vi "modSingle.vi"(0 "signal":fxp<+,18,0>, 1 "Parameters":T1, 2 "Enable":bool, 11 "triangleOffset":fxp<+,19,1>) -> (4 "output":T2)   [LabVIEW 2017, in "BuckBoost.lvlib"]
uses:
  BuckBoost.lvlib
  modOutput.ctl
  modParameters.ctl
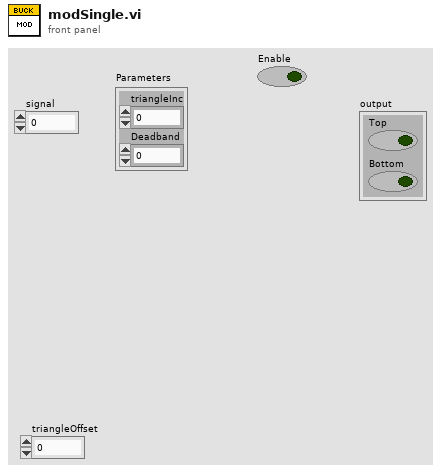
[diagram p1: front panel]
types:
  T1 = typedef "BuckBoost.lvlib/modParameters.ctl" = cluster{"triangleInc":fxp<+,18,0>, "Deadband":u16}
  T2 = typedef "BuckBoost.lvlib/modOutput.ctl" = cluster{"Top":bool, "Bottom":bool}
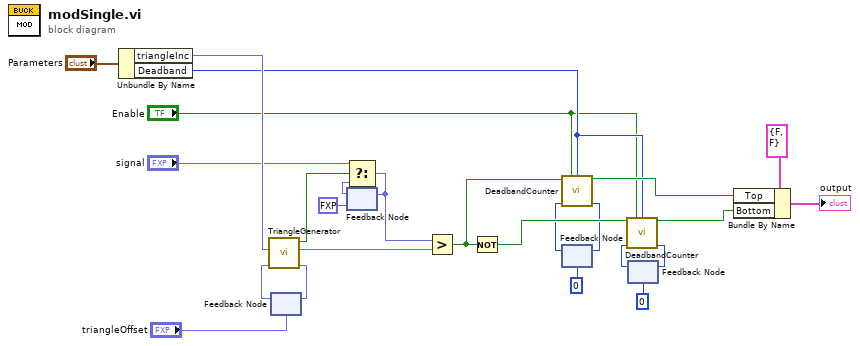
[diagram p0: block diagram]
diagram:
  n1 = Unbundle By Name("Parameters") -> ("triangleInc"=w17:fxp<+,18,0>, "Deadband"=w16:u16)
  n2 = feedback #1("triangleOffset") -> (w3:fxp<+,19,1>)
  n3 = call "TriangleGenerator.vi"("stateIn"=w3, "triangleInc"=w17) -> ("stateOut"=w4:fxp<+,19,1>, "triangle"=w19:fxp<+,18,0>, "cycleComplete"=w14:bool)  [unwired: 7 in]
  n4 = feedback-in #1(w4) -> ()
  n5 = feedback #2(fxp<+,18,0> 0.0 ("signal")) -> (w13:fxp<+,18,0>)
  n6 = Select(t="signal", s=w14, f=w13) -> (s? t:f=w11:fxp<+,18,0>)
  n7 = feedback-in #2(w11) -> ()
  n8 = Greater?(x=w11, y=w19) -> (0:w20:bool)
  n9 = Not(x=w20) -> (.not. x?=w21:bool)
  n10 = feedback #3(u16 0 ("stateOut")) -> (w5:u16)
  n11 = call "DeadbandCounter.vi"("Input"=w20, "Enable"="Enable", "Deadtime"=w16, "stateIn"=w5) -> ("Output"=w23:bool, "stateOut"=w6:u16)  [unwired: 10 in]
  n12 = feedback-in #3(w6) -> ()
  n13 = feedback #4(u16 0 ("stateOut")) -> (w9:u16)
  n14 = call "DeadbandCounter.vi"("Input"=w21, "Enable"="Enable", "Deadtime"=w16, "stateIn"=w9) -> ("Output"=w24:bool, "stateOut"=w10:u16)  [unwired: 10 in]
  n15 = feedback-in #4(w10) -> ()
  n16 = Bundle By Name(cluster=T2 {"Top"=FALSE, "Bottom"=FALSE}, "Top"=w23, "Bottom"=w24) -> (→"output":T2)
